vi "mupLib example.vi"() -> ()   [LabVIEW 2015]
uses:
  mupLib/mupCheckError.vi
  <vilib>/Utility/error.llb/Error Cluster From Error Code.vi
  muParser.lvlib
panel:
  out "Array":dbl[](array[numeric])
  in  "c":dbl
  in  "szExpr":string="a*x^2+b*x+c"
  in  "x":dbl
  in  "b":dbl
  in  "a":dbl
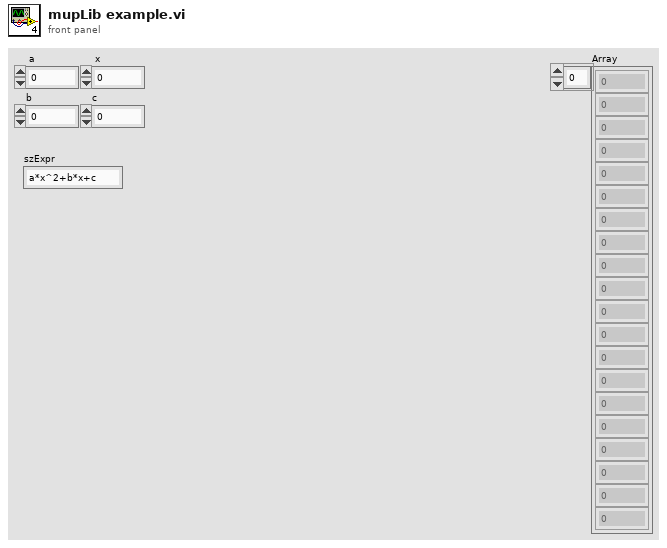
[diagram p1: front panel]
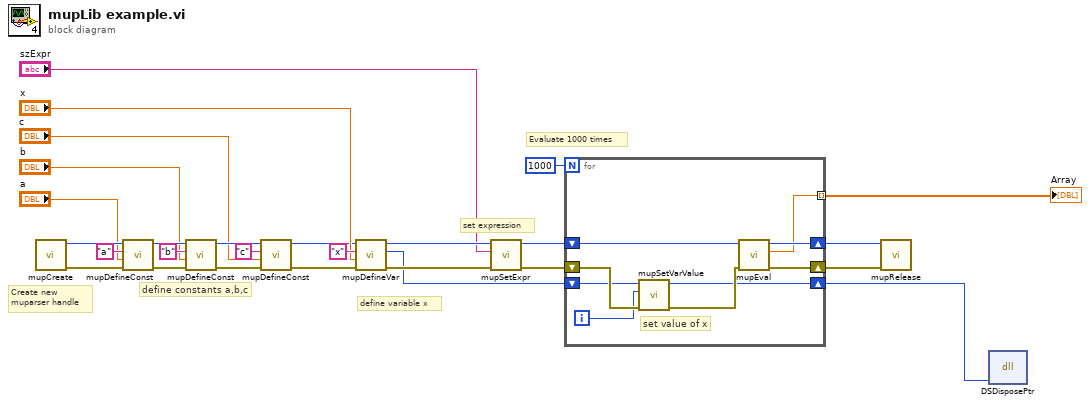
[diagram p0: block diagram]
diagram:
  # "Evaluate 1000 times"
  # "set expression"
  # "define variable x"
  # "define constants a,b,c"
  # "Create new\nmuparser handle"
  n1 = call "mupCreate.vi"() -> ("error out"=w26:errorcluster, "hParser"=w27:u64)  [unwired: 10 in]
  n2 = call "mupDefineConst.vi"("error in (no error)"=w26, "Value"="a", "constName"="a", "hParser in"=w27) -> ("error out"=w21:errorcluster, "hParser out"=w22:u64)  [unwired: 6 in]
  n3 = call "mupDefineConst.vi"("error in (no error)"=w21, "Value"="b", "constName"="b", "hParser in"=w22) -> ("error out"=w12:errorcluster, "hParser out"=w13:u64)  [unwired: 6 in]
  n4 = call "mupDefineConst.vi"("error in (no error)"=w12, "Value"="c", "constName"="c", "hParser in"=w13) -> ("error out"=w10:errorcluster, "hParser out"=w9:u64)  [unwired: 6 in]
  n5 = call "mupDefineVar.vi"("error in (no error)"=w10, "initValue"="x", "varName"="x", "hParser in"=w9) -> ("error out"=w15:errorcluster, "varAddr"=w5:u64, "hParser out"=w17:u64)  [unwired: 5 in]
  n6 = call "mupSetExpr.vi"("error in (no error)"=w15, "szExpr"="szExpr", "hParser in"=w17) -> ("error out"=w7:errorcluster, "hParser out"=w8:u64)  [unwired: 7 in]
  n7 = for {
    N: 1000 -> [_]
    shift-right: [w30] -> w2
    shift-left: w8 -> [w33]
    shift-right: [w31] -> w1
    shift-left: w7 -> [w36]
    tunnel: [w29] -> w6 mode=indexing
    shift-right: [w28] -> w4
    shift-left: w5 -> [w35]
    i -> [w34]
    # "set value of x"
    n8 = call "mupSetVarValue.vi"("error in (no error)"=w36, "varValue"=w34, "varPtr in"=w35) -> ("error out"=w32:errorcluster, "varPtr out"=w28:u64)  [unwired: 7 in]
    n9 = call "mupEval.vi"("error in (no error)"=w32, "hParser in"=w33) -> ("error out"=w31:errorcluster, "result"=w29:dbl, "hParser out"=w30:u64)  [unwired: 7 in]
  }
  "Array" <- w6
  n10 = call "mupRelease.vi"("error in (no error)"=w1, "hParser"=w2) -> ()  [unwired: 9 in, 1 out]
  n11 = dll-call lib="LabVIEW" fn="DSDisposePtr"("ptr"=w4) -> ()  [unwired: 5 in, 2 out]
